vi "Write Num1.lvclass.vi"(8 "error in (no error)":errorcluster, 10 "Num1.lvclass":refnum<class "Num1.lvclass">, 11 "POffset.lvclass in":refnum<class "POffset.lvclass">) -> (0 "error out":errorcluster, 3 "POffset.lvclass out":refnum<class "POffset.lvclass">)   [LabVIEW 2009, in "POffset.lvclass"]
uses:
  POffset.lvclass
  OffsetCommands/OffsetDef/Num1/Num1.lvclass
  POffset.lvclass/POffset.ctl
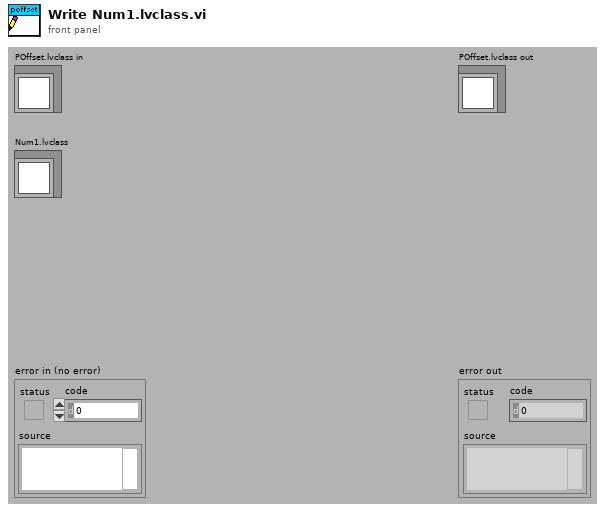
[diagram p1: front panel]
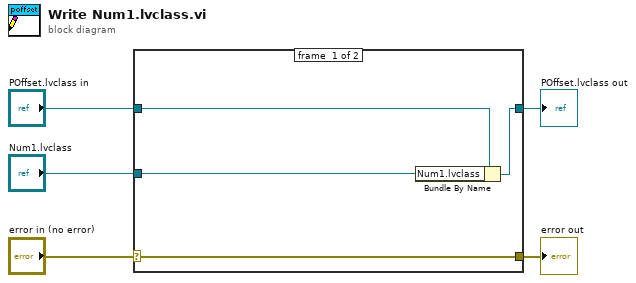
[diagram p0: block diagram]
diagram:
  n1 = case shown="No Error" "error in (no error)" {
    selector: "error in (no error)" -> [w9 w10]
    tunnel: [w9 w10] -> w4
    tunnel: [w7 w11] -> w2
    tunnel: "POffset.lvclass in" -> [w8 w11]
    tunnel: "Num1.lvclass" -> [w6 _]
    frame #0 {
      n2 = Bundle By Name(cluster=w8, "Num1.lvclass"=w6) -> (w7:refnum<class "POffset.lvclass">)
    }
    frame #1 {
    }
  }
  "error out" <- w4
  "POffset.lvclass out" <- w2
